vi "Creator Attributes.vi"(11 "Actor in":refnum<class "Actor.lvclass">) -> (2 "Creator Attributes":T1)   [LabVIEW 2021, in "jettl.lvlib" / "Actor.lvlib" / "Actor.lvclass"]
uses:
  Actor.lvclass
  Msg/Msg.lvclass
  Implemented Msgs.ctl
  Actor.lvlib
  Attributes.ctl
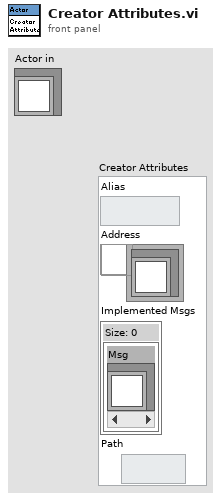
[diagram p1: front panel]
types:
  T1 = typedef "jettl.lvlib/Actor.lvlib/Attributes.ctl" = cluster{"Alias":string, "Address":refnum<user-event>, "Implemented Msgs":T2, "Path":path}
  T2 = typedef "jettl.lvlib/Actor.lvlib/Implemented Msgs.ctl" = set{refnum<class "Msg.lvclass">}
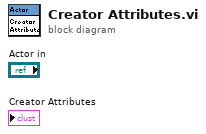
[diagram p0: block diagram]
diagram:
